vi "Read.vi"(8 "error in (no error)":errorcluster, 9 "Starting independent variable":dbl, 10 "Current independent variable":dbl, 11 "LCD Reader in":refnum<class "LCD Reader.lvclass">) -> (0 "error out":errorcluster, 2 "Data Channels":T1, 3 "LCD Reader out":refnum<class "LCD Reader.lvclass">)   [LabVIEW 2009, in "LCD Reader.lvclass"]
doc: "Prepare for read, wait the time delay, and take data from up to 4 channels."
uses:
  LCD Reader.lvclass
  Instruments/Utility Classes/Readable/Data Channels.ctl
  Instruments/Utility Classes/Readable/Data Channel.ctl
  Instruments/Utility Classes/Readable/Data Point.ctl
  Instruments/LCD/LCD Retarder.lvclass
  LCD Reader.lvclass/LCD Reader.ctl
  Reader/Reader.lvclass
  Instruments/Utility Classes/Readable/Readable.lvclass
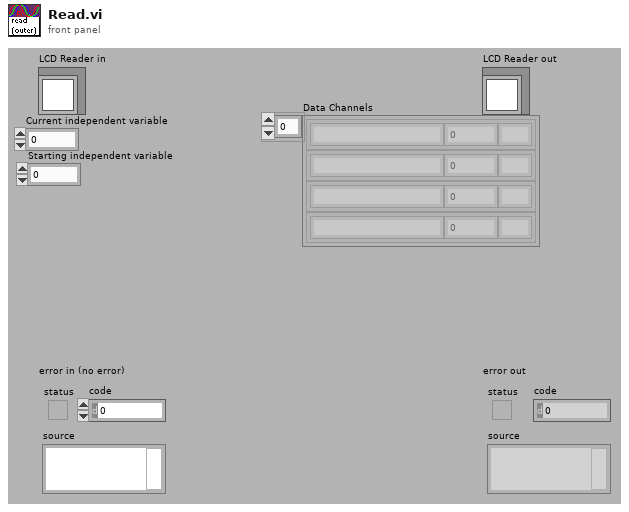
[diagram p1: front panel]
types:
  T1 = typedef "Readable.lvclass/Data Channels.ctl" = T2[]
  T2 = typedef "Readable.lvclass/Data Channel.ctl" = cluster{"Name":string, "Data Point":T3, "Unit":string}
  T3 = typedef "Readable.lvclass/Data Point.ctl" = dbl
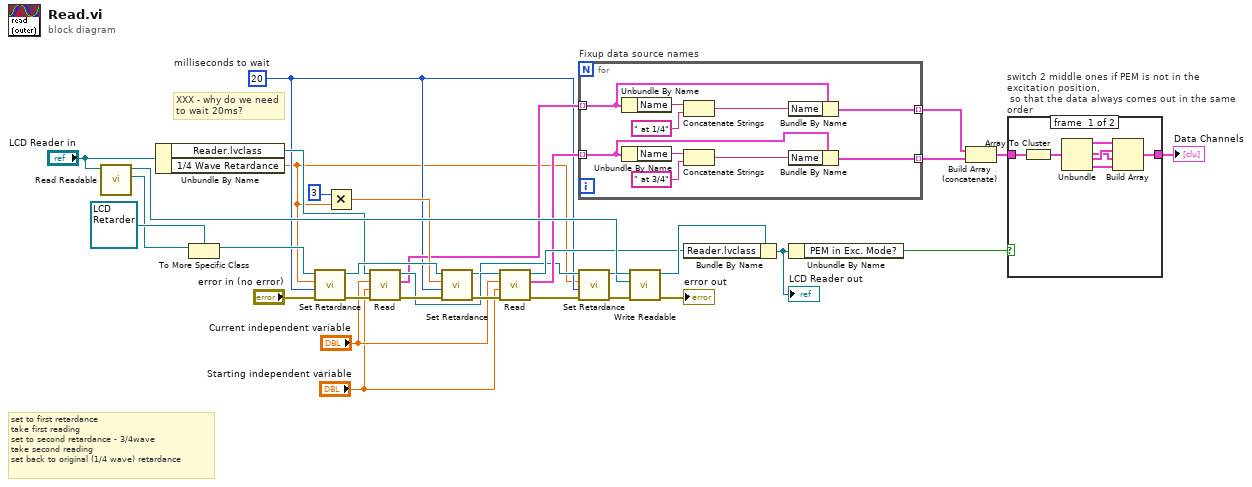
[diagram p0: block diagram]
diagram:
  w4 = u32 20  # milliseconds to wait
  # "XXX - why do we need\nto wait 20ms?"
  # "set to first retardance\ntake first reading\nset to second retardance - 3/4wave\ntake second reading\nset back to original (1/4 wave) retardance"
  n1 = call-dynamic "Read Readable.vi"("Reader.lvclass in"="LCD Reader in") -> ("Readable.lvclass"=w29:refnum<class "Readable.lvclass">, "Reader.lvclass out"=w25:refnum<class "LCD Reader.lvclass">)  [unwired: 1 in, 8 out]
  n2 = Unbundle By Name("LCD Reader in") -> ("Reader.lvclass"=w21:refnum<class "Reader.lvclass">, "1/4 Wave Retardance"=w1:dbl[unit])
  n3 = To More Specific Class(target class=refnum<class "LCD Retarder.lvclass"> refnum ("LCD Retarder.lvclass"), reference=w29) -> (specific class reference=w28:refnum<class "LCD Retarder.lvclass">)  [unwired: 1 in, 1 out]
  n4 = call "Set Retardance.vi"("errorIN"="error in (no error)", "milliseconds to wait (0)"=w4, "Retardance"=w1, "LCD in"=w28) -> ("errorOUT"=w27:errorcluster, "LCD out"=w31:refnum<class "LCD Retarder.lvclass">)  [unwired: 6 out]
  n5 = Multiply(x=3, y=w1) -> (x*y=w12:dbl[unit])
  n6 = call-dynamic "Read.vi"("error in (no error)"=w27, "Starting independent variable"="Starting independent variable", "Current independent variable"="Current independent variable", "Reader in"=w21) -> ("error out"=w26:errorcluster, "Data Channels"=w11:T1, "Reader out"=w23:refnum<class "Reader.lvclass">)  [unwired: 5 out]
  n7 = call "Set Retardance.vi"("errorIN"=w26, "milliseconds to wait (0)"=w4, "Retardance"=w12, "LCD in"=w31) -> ("errorOUT"=w24:errorcluster, "LCD out"=w7:refnum<class "LCD Retarder.lvclass">)  [unwired: 6 out]
  n8 = call-dynamic "Read.vi"("error in (no error)"=w24, "Starting independent variable"="Starting independent variable", "Current independent variable"="Current independent variable", "Reader in"=w23) -> ("error out"=w5:errorcluster, "Data Channels"=w10:T1, "Reader out"=w19:refnum<class "Reader.lvclass">)  [unwired: 5 out]
  n9 = for "Fixup data source names" {
    tunnel: w11 -> [w36] mode=indexing
    tunnel: w10 -> [w39] mode=indexing
    tunnel: [w38] -> w9 mode=indexing
    tunnel: [w34] -> w8 mode=indexing
    n10 = Unbundle By Name(w36) -> ("Name"=w40:string)
    n11 = Unbundle By Name(w39) -> ("Name"=w43:string)
    n12 = Concatenate Strings(w40, " at 1/4" ("string")) -> (w35:string)
    n13 = Concatenate Strings(w43, " at 3/4" ("string")) -> (w37:string)
    n14 = Bundle By Name(cluster=w36, "Name"=w35) -> (w34:T2)
    n15 = Bundle By Name(cluster=w39, "Name"=w37) -> (w38:T2)
  }
  n16 = call "Set Retardance.vi"("errorIN"=w5, "milliseconds to wait (0)"=w4, "Retardance"=w1, "LCD in"=w7) -> ("errorOUT"=w3:errorcluster, "LCD out"=w6:refnum<class "LCD Retarder.lvclass">)  [unwired: 6 out]
  n17 = call-dynamic "Write Readable.vi"("error in (no error)"=w3, "Readable.lvclass"=w6, "Reader.lvclass in"=w25) -> ("error out"=→"error out":errorcluster, "Reader.lvclass out"=w20:refnum<class "LCD Reader.lvclass">)  [unwired: 7 out]
  n18 = Bundle By Name(cluster=w20, "Reader.lvclass"=w19) -> (w14:refnum<class "LCD Reader.lvclass">)
  "LCD Reader out" <- w14
  n19 = Unbundle By Name(w14) -> ("PEM in Exc. Mode?"=w13:bool)
  n20 = Build Array (concatenate)(w8, w9) -> (w33:T2[])
  n21 = case "switch 2 middle ones if PEM is not in the excitation position,\n so that the data always comes out in the same order" shown="False" w13 {
    tunnel: w33 -> [w50 w51]
    tunnel: [w46 w51] -> w16
    frame #0 {
      n22 = Array To Cluster(array=w50) -> (cluster=w49:cluster{"[0]":T2, "[1]":T2, "[2]":T2, "[3]":T2})
      n23 = Unbundle(w49) -> ("[0]"=w48:T2, "[1]"=w44:T2, "[2]"=w45:T2, "[3]"=w47:T2)
      n24 = Build Array(w48, w45, w44, w47) -> (w46:T2[])
    }
    frame #1 {
    }
  }
  "Data Channels" <- w16
